vi "LVClass_CorrectionDataManager SetActuatorPrefs.vi"(0 "CorrectionDataManager in":refnum<class "CorrectionDataManager.lvclass">, 5 "Index of actuator":dbl, 7 "Actuator state":T1, 11 "error in (no error)":errorcluster) -> (4 "CorrectionDataManager out":refnum<class "CorrectionDataManager.lvclass">, 8 "New data Need":bool, 15 "error out":errorcluster)   [LabVIEW 2020, in "CorrectionDataManager.lvclass"]
uses:
  CorrectionDataManager.lvclass
  Wavefront Corrector states - ONE.ctl
  CorrectionDataManager.lvclass/CorrectionDataManager.ctl
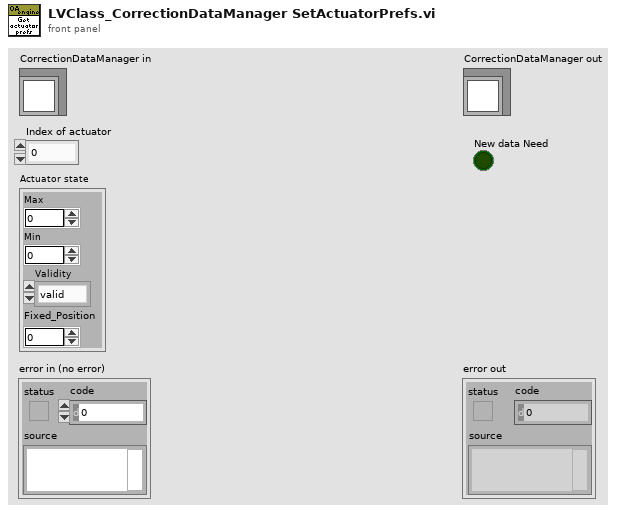
[diagram p1: front panel]
types:
  T1 = typedef "Wavefront Corrector states - ONE.ctl" = cluster{"Max":sgl, "Min":sgl, "Validity":enum16{"valid", "fixed", "invalid"}, "Fixed_Position":sgl}
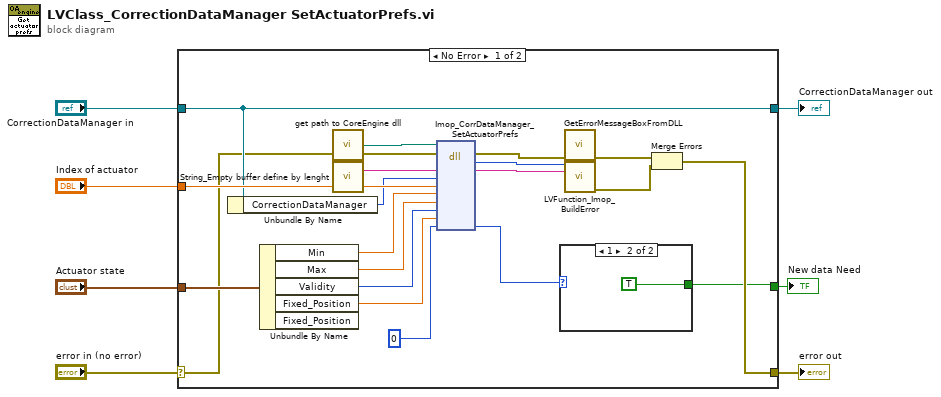
[diagram p0: block diagram]
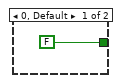
[diagram p2: hidden frame]
diagram:
  n1 = case shown="No Error" "error in (no error)" {
    selector: "error in (no error)" -> [w12 w31]
    tunnel: [w11 w31] -> w6
    tunnel: [w19 w30] -> w4
    tunnel: "CorrectionDataManager in" -> [w19 w30]
    tunnel: "Index of actuator" -> [w20 _]
    tunnel: "Actuator state" -> [w17 _]
    tunnel: [w8 _] -> w1
    frame No Error {
      n2 = Unbundle By Name(w19) -> ("CorrectionDataManager"=w18:i32)
      n3 = Unbundle By Name(w17) -> ("Min"=w16:sgl, "Max"=w15:sgl, "Validity"=w14:enum16{"valid", "fixed", "invalid"}, "Fixed_Position"=w13:sgl)  [unwired: 1 out]
      n4 = call "get path to CoreEngine dll.vi"() -> ("path to c_interface_vc100.dll"=w25:path)  [unwired: 12 in, 3 out]
      n5 = call "String_Empty buffer define by lenght.vi"() -> ("Empty buffer"=w24:string)  [unwired: 1 in]
      n6 = dll-call lib="D:/FLE/0.Code/CoreEngine4_Suite/LV2011_interface/DLLs/c_interface_vc100.dll" fn="Imop_CorrDataManager_SetActuatorPrefs"(path in=w25, error in=w12, "Message"=w24, "CorrectionDataManager"=w18, "Actuator index"=w20, "Min"=w16, "Max"=w15, "Validity"=w14, "Fixed position"=w13, "New data needed"=u8 0) -> (error out=w23:errorcluster, "return type"=w22:i32, "Message"=w21:string, "New data needed"=w9:u8)  [unwired: 7 in, 1 out]
      n7 = case shown="1" w9 {
        tunnel: [FALSE TRUE] -> w8
        frame 0, Default {
        }
        frame 1 {
        }
      }
      n8 = call "GetErrorMessageBoxFromDLL.vi"("error IN"=w23) -> ("error OUT"=w27:errorcluster)  [unwired: 10 in]
      n9 = call "LVFunction_Imop_BuildError.vi"("code"=w22, "String to Prepend to source (\"\")"=w21) -> ("error out"=w26:errorcluster)  [unwired: 13 in]
      n10 = Merge Errors(w27, w26) -> (w11:errorcluster)
    }
    frame Error {
    }
  }
  "error out" <- w6
  "CorrectionDataManager out" <- w4
  "New data Need" <- w1
